vi "Trigger.vi"(5 "Trigger Settings":T1, 8 "error in":errorcluster {"code" format="%.0x"}, 9 "Vertical range Channel B":dbl, 10 "Vertical range Channel A":dbl, 11 "instrument handle":refnum<k15> caption="instrument handle in") -> (0 "error out":errorcluster {"code" format="%.0x"}, 2 "Trigger Level":dbl, 3 "instrument handle":refnum<k15> caption="instrument handle out")   [LabVIEW 2011]
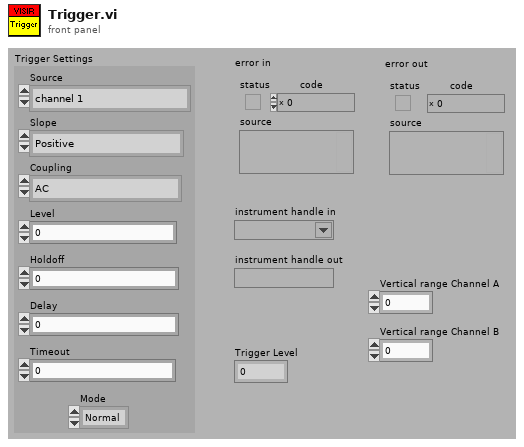
[diagram p1: front panel]
types:
  T1 = cluster{"Source":enum8{"channel 1", "channel 2", "Imediate", "External trigger"}, "Slope":enum8{"Positive", "Negative"}, "Coupling":enum8{"AC", "DC"}, "Level":dbl, "Holdoff":dbl, "Delay":dbl, "Timeout":dbl, "Mode":enum8{"Normal", "Auto", "Auto Level"}}
  T2 = enum8{"channel 1", "channel 2", "Imediate", "External trigger"}
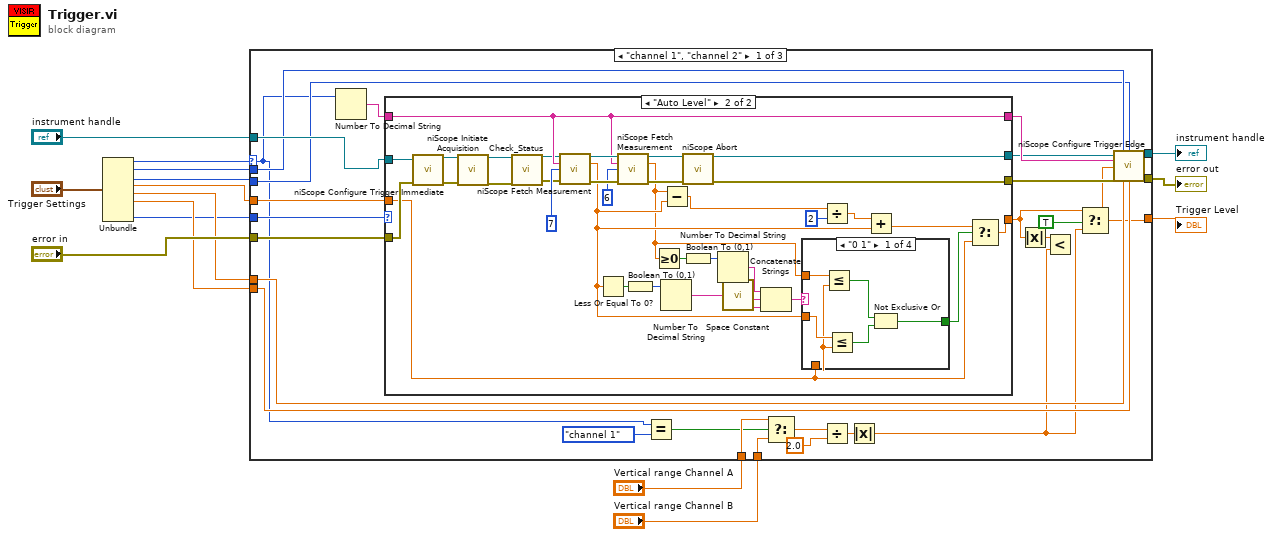
[diagram p0: block diagram]
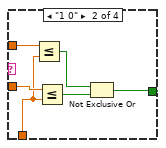
[diagram p3: hidden frame]
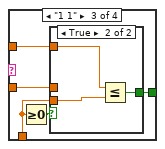
[diagram p4: hidden frame]
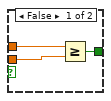
[diagram p5: hidden frame]
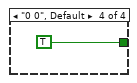
[diagram p6: hidden frame]
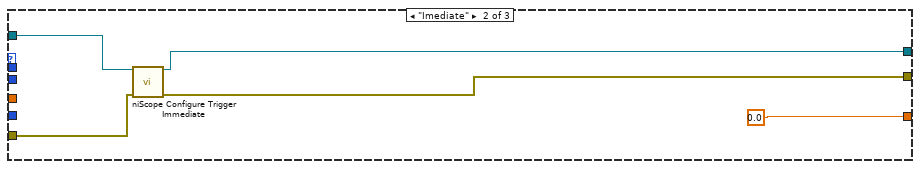
[diagram p7: hidden frame]
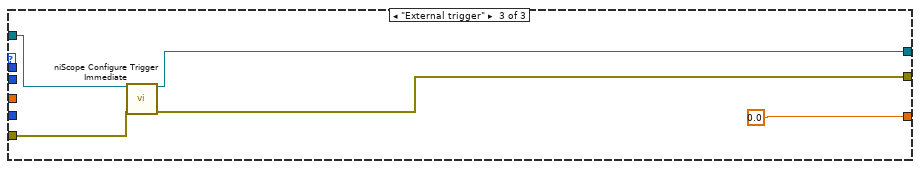
[diagram p8: hidden frame]
diagram:
  n1 = Unbundle("Trigger Settings") -> ("Source"=w3:T2, "Slope"=w11:enum8{"Positive", "Negative"}, "Coupling"=w5:enum8{"AC", "DC"}, "Level"=w10:dbl, "Holdoff"=w9:dbl, "Delay"=w8:dbl, "Mode"=w6:enum8{"Normal", "Auto", "Auto Level"})  [unwired: 1 out]
  n2 = case shown="\"channel 1\", \"channel 2\"" w3 {
    selector: w3 -> [w23 _ _]
    tunnel: "error in" -> [w40 w109 w112]
    tunnel: "instrument handle" -> [w41 w108 w111]
    tunnel: [w35 w107 w114] -> w12
    tunnel: [w34 w106 w113] -> w7
    tunnel: w11 -> [w39 _ _]
    tunnel: w5 -> [w37 _ _]
    tunnel: w10 -> [w33 _ _]
    tunnel: w9 -> [w38 _ _]
    tunnel: w8 -> [w36 _ _]
    tunnel: w6 -> [w42 _ _]
    tunnel: [w17 0.0 0.0] -> w4
    tunnel: "Vertical range Channel A" -> [w25 _ _]
    tunnel: "Vertical range Channel B" -> [w24 _ _]
    frame "channel 1", "channel 2" {
      n3 = Number To Decimal String(number=w23) -> (decimal integer string=w32:string)  [unwired: 1 in]
      n4 = case shown="\"Auto Level\"" w42 {
        tunnel: w41 -> [w44 w80]
        tunnel: w40 -> [w45 w79]
        tunnel: w32 -> [w43 w71]
        tunnel: [w46 w62] -> w19
        tunnel: [w44 w69] -> w30
        tunnel: [w45 w68] -> w29
        tunnel: w33 -> [w46 w50]
        tunnel: [w43 w71] -> w31
        frame "Normal", "Auto", Default {
        }
        frame "Auto Level" {
          n5 = call <instrlib>:"niScope Configure Trigger Immediate.vi"("instrument handle"=w80, "error in"=w79) -> ("instrument handle out"=w78:refnum<k15>, "error out"=w77:errorcluster)  [unwired: 12 in]
          n6 = call <instrlib>:"niScope Initiate Acquisition.vi"("instrument handle"=w78, "error in"=w77) -> ("instrument handle out"=w66:refnum<k15>, "error out"=w65:errorcluster)  [unwired: 12 in]
          n7 = call "Check_Status.vi"("error in"=w65, "instrument handle in"=w66) -> ("error out"=w63:errorcluster, "instrument handle out"=w64:refnum<k15>)
          n8 = call <instrlib>:"niScope Fetch Measurement.vi"("instrument handle"=w64, "channels"=w71, "scalar measurement"=7, "error in"=w63) -> ("instrument handle out"=w74:refnum<k15>, "result"=w49:dbl, "error out"=w73:errorcluster)  [unwired: 9 in]
          n9 = Less Or Equal To 0?(x=w49) -> (x <= 0?=w57:bool)
          n10 = call <instrlib>:"niScope Fetch Measurement.vi"("instrument handle"=w74, "channels"=w71, "scalar measurement"=6, "error in"=w73) -> ("instrument handle out"=w70:refnum<k15>, "result"=w48:dbl, "error out"=w67:errorcluster)  [unwired: 9 in]
          n11 = Boolean To (0,1)(Boolean=w57) -> (0, 1=w55:i16)
          n12 = Greater Or Equal To 0?(x=w48) -> (x >= 0?=w58:bool)
          n13 = Number To Decimal String(number=w55) -> (decimal integer string=w52:string)  [unwired: 1 in]
          n14 = Subtract(x=w48, y=w49) -> (x-y=w61:dbl)
          n15 = call <instrlib>:"niScope Abort.vi"("instrument handle"=w70, "error in"=w67) -> ("instrument handle out"=w69:refnum<k15>, "error out"=w68:errorcluster)  [unwired: 12 in]
          n16 = Boolean To (0,1)(Boolean=w58) -> (0, 1=w56:i16)
          n17 = Number To Decimal String(number=w56) -> (decimal integer string=w53:string)  [unwired: 1 in]
          n18 = call <vilib>:"Space Constant.vi"() -> ("String"=w51:string)
          n19 = Concatenate Strings(w53, w51, w52) -> (w54:string)
          n20 = case shown="\"0 1\"" w54 {
            tunnel: w50 -> [w82 w90 w95 _]
            tunnel: w49 -> [w83 w92 w93 _]
            tunnel: w48 -> [w84 w91 w96 _]
            tunnel: [w81 w87 w94 TRUE] -> w47
            frame "0 1" {
              n21 = Less Or Equal?(x=w84, y=w82) -> (x <= y?=w86:bool)
              n22 = Less Or Equal?(x=w83, y=w82) -> (x <= y?=w85:bool)
              n23 = Not Exclusive Or(1:w85, 2:w86) -> (0:w81:bool)
            }
            frame "1 0" {
              n24 = Less Or Equal?(x=w91, y=w90) -> (x <= y?=w89:bool)
              n25 = Less Or Equal?(x=w92, y=w90) -> (x <= y?=w88:bool)
              n26 = Not Exclusive Or(1:w88, 2:w89) -> (0:w87:bool)
            }
            frame "1 1" {
              n27 = Greater Or Equal To 0?(x=w95) -> (x >= 0?=w97:bool)
              n28 = case shown="True" w97 {
                tunnel: w96 -> [_ w103]
                tunnel: w95 -> [w99 w102]
                tunnel: [w98 w101] -> w94
                tunnel: w93 -> [w100 _]
                frame False {
                  n29 = Greater Or Equal?(x=w100, y=w99) -> (x >= y?=w98:bool)
                }
                frame True {
                  n30 = Less Or Equal?(x=w103, y=w102) -> (x <= y?=w101:bool)
                }
              }
            }
            frame "0 0", Default {
            }
          }
          n31 = Divide(x=w61, y=i8 2) -> (x/y=w60:dbl)
          n32 = Add(x=w60, y=w49) -> (x+y=w59:dbl)
          n33 = Select(t=w59, s=w47, f=w50) -> (s? t:f=w62:dbl)
        }
      }
      n34 = Equal?(x=w23, y=T2."channel 1") -> (x = y?=w21:bool)
      n35 = Select(t=w25, s=w21, f=w24) -> (s? t:f=w20:dbl)
      n36 = Divide(x=w20, y=2.0) -> (x/y=w28:dbl)
      n37 = Absolute Value(x=w28) -> (abs(x)=w18:dbl)
      n38 = Absolute Value(x=w19) -> (abs(x)=w26:dbl)
      n39 = Less?(x=w26, y=w18) -> ()  [unwired: 1 out]
      n40 = Select(t=w19, s=TRUE, f=w18) -> (s? t:f=w17:dbl)
      n41 = call <instrlib>:"niScope Configure Trigger Edge.vi"("instrument handle"=w30, "trigger slope"=w39, "trigger coupling"=w37, "trigger source"=w31, "trigger level"=w17, "error in"=w29, "trigger holdoff"=w38, "trigger delay"=w36) -> ("instrument handle out"=w35:refnum<k15>, "error out"=w34:errorcluster)  [unwired: 6 in]
    }
    frame "Imediate" {
      n42 = call <instrlib>:"niScope Configure Trigger Immediate.vi"("instrument handle"=w108, "error in"=w109) -> ("instrument handle out"=w107:refnum<k15>, "error out"=w106:errorcluster)  [unwired: 12 in]
    }
    frame "External trigger" {
      n43 = call <instrlib>:"niScope Configure Trigger Immediate.vi"("instrument handle"=w111, "error in"=w112) -> ("instrument handle out"=w114:refnum<k15>, "error out"=w113:errorcluster)  [unwired: 12 in]
    }
  }
  "error out" <- w7
  "instrument handle" <- w12
  "Trigger Level" <- w4
